vi "CreateObject.vi"(8 "error in (no error)":errorcluster, 10 "Bounds":T1) -> (0 "error out":errorcluster, 3 "DisplayWindow out":refnum<class "DisplayWindow.lvclass">)   [LabVIEW 2016, in "DisplayWindow.lvlib" / "DisplayWindow.lvclass"]
uses:
  DisplayWindow.lvclass
  <vilib>/Utility/miscctls.llb/LVRectTypeDef.ctl
  DisplayWindow.lvclass/DisplayWindow.ctl
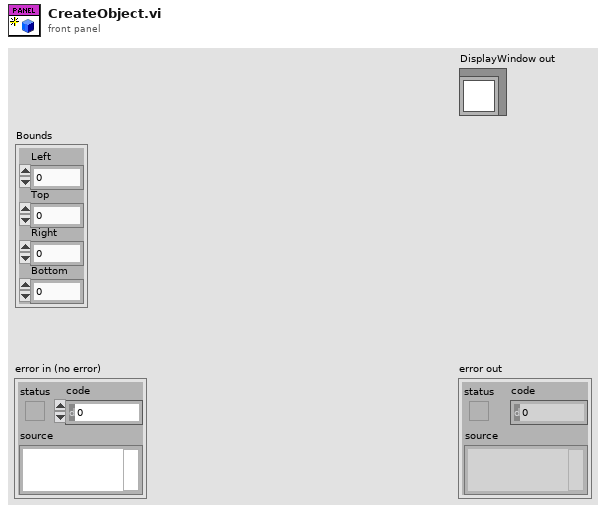
[diagram p1: front panel]
types:
  T1 = typedef "LVRectTypeDef.ctl" = cluster{"Left":i16, "Top":i16, "Right":i16, "Bottom":i16}
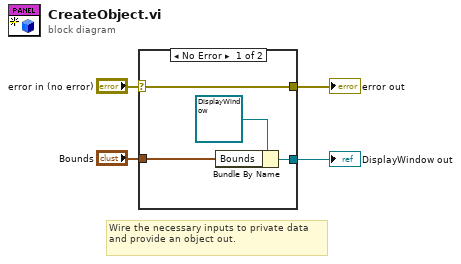
[diagram p0: block diagram]
diagram:
  # "Wire the necessary inputs to private data and provide an object out."
  n1 = case shown="No Error" "error in (no error)" {
    selector: "error in (no error)" -> [w8 w9]
    tunnel: [w8 w9] -> w3
    tunnel: [w6 _] -> w2
    tunnel: "Bounds" -> [w5 _]
    frame No Error {
      n2 = Bundle By Name(cluster=refnum<class "DisplayWindow.lvclass"> refnum ("DisplayWindow.lvlib:DisplayWindow.lvclass"), "Bounds"=w5) -> (w6:refnum<class "DisplayWindow.lvclass">)
    }
    frame Error {
    }
  }
  "error out" <- w3
  "DisplayWindow out" <- w2
